vi "HelpDialog.vi"(8 "REPL Name":string, 9 "CodeRef":refnum<vi>, 11 "Microprocessor in":T1) -> (3 "Microprocessor out":T1)   [LabVIEW 2016]
uses:
  <userlib>/MicroPython/VIs/ColorText/Code.xctl
  <vilib>/Platform/browser.llb/Open URL in Default Browser (string).vi
panel:
  in  "Examples":string(tree)
  in  "Processor":u16(ring) items=["Generic", "Huzzah", "MicroBit", "OpenMV", "Pololu", "PyBoard", "PyCom"]
  in  "Copy":bool
  out "Code":string(xcontrol)
  # "If things do not work:\n1. check that you have NI-VISA installed"
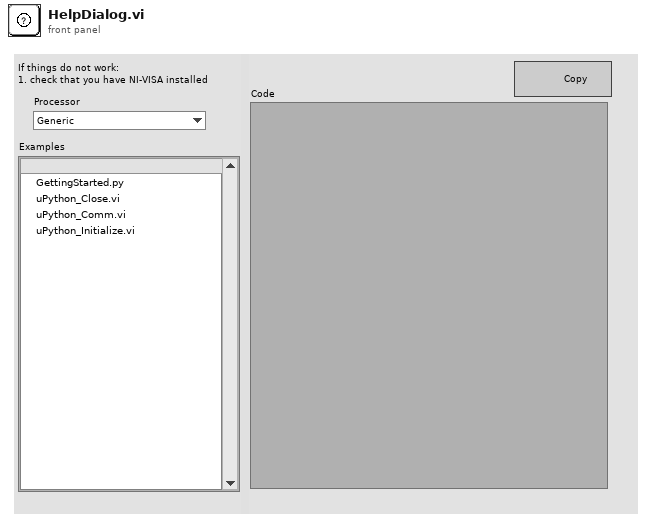
[diagram p1: front panel]
types:
  T1 = cluster{"VISA Refnum in":refnum<visa-resource-name>, "Python Code":string}
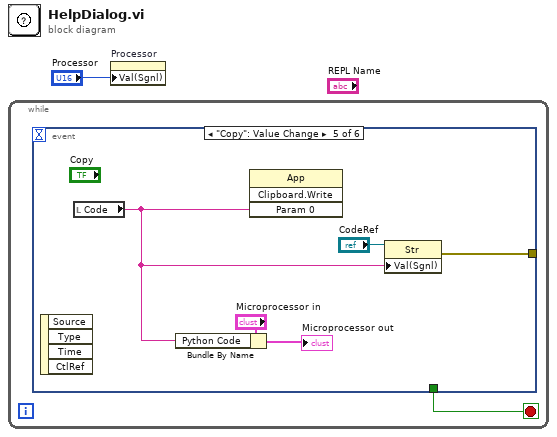
[diagram p0: block diagram]
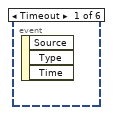
[diagram p2: hidden frame]
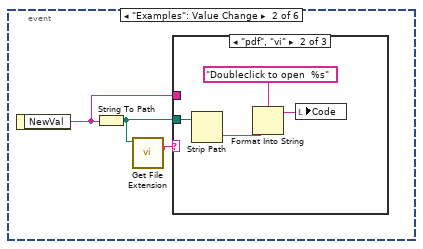
[diagram p3: hidden frame]
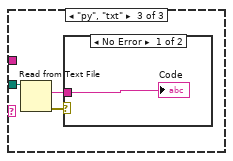
[diagram p5: hidden frame]
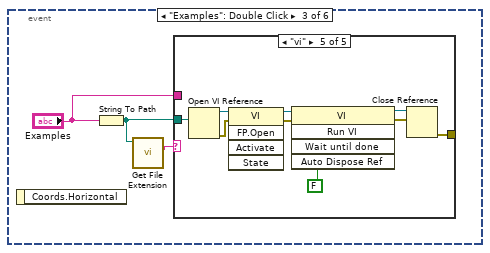
[diagram p7: hidden frame]
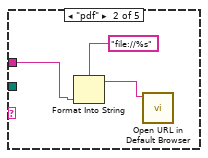
[diagram p9: hidden frame]
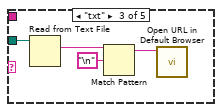
[diagram p10: hidden frame]
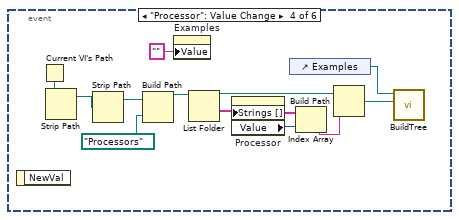
[diagram p12: hidden frame]
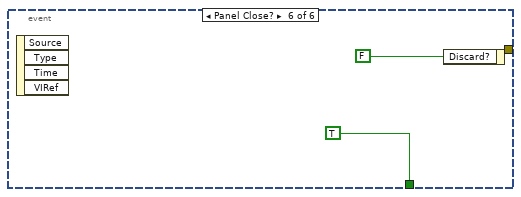
[diagram p13: hidden frame]
diagram:
  n1 = while {
    stop <- w2 stop-if-true
    n2 = event shown="[4] \"Copy\": Value Change" {
      selector: _ -> [_ _ _ _ _ _]
      dyn-events: _ -> [_ _ _ _ _ _]
      timeout: _ -> [_ _ _ _ _ _]
      tunnel: [_ _ _ _ _ TRUE ("Discard?")] -> w2
      tunnel: [_ _ _ _ w46 _] -> _
      event Timeout {
        n3 = event-data() -> ()  [unwired: 1 in, 3 out]
      }
      event "Examples": Value Change {
        n4 = event-data() -> ("NewVal"=w3:string)  [unwired: 1 in]
        n5 = String To Path(string=w3) -> (path=w5:path)
        n6 = call <vilib>:"Get File Extension.vi"("file"=w5) -> ("lowercase file extension"=w4:string)  [unwired: 6 in, 4 out]
        n7 = case shown="\"pdf\", \"vi\"" w4 {
          tunnel: w5 -> [_ w7 w10]
          tunnel: w3 -> [_ _ _]
          frame Default {
          }
          frame "pdf", "vi" {
            n8 = Strip Path(path=w7) -> (name=w6:string)  [unwired: 1 out]
            n9 = Format Into String(format string="Doubleclick to open  %s", w6) -> (resulting string=w8:string)  [unwired: 2 in, 1 out]
            n10 = local write "Code"(w8) -> ()
          }
          frame "py", "txt" {
            n11 = Read from Text File(file (use dialog)=w10) -> (text=w12:string, error out=w11:errorcluster)  [unwired: 3 in, 2 out]
            n12 = case shown="No Error" w11 {
              tunnel: w12 -> [w13 _]
              frame No Error {
                "Code" <- w13
              }
              frame Error {
              }
            }
          }
        }
      }
      event "Examples": Double Click {
        n13 = event-data() -> ()  [unwired: 1 in, 1 out]
        n14 = String To Path(string="Examples") -> (path=w16:path)
        n15 = call <vilib>:"Get File Extension.vi"("file"=w16) -> ("lowercase file extension"=w15:string)  [unwired: 6 in, 4 out]
        n16 = case shown="\"vi\"" w15 {
          tunnel: w16 -> [_ _ w23 _ w32]
          tunnel: "Examples" -> [_ w18 _ _ _]
          tunnel: [_ _ _ _ w29] -> _
          frame Default {
          }
          frame "pdf" {
            n17 = Format Into String(format string="file://%s", w18) -> (resulting string=w17:string)  [unwired: 2 in, 1 out]
            n18 = call-poly <vilib>:"Open URL in Default Browser.vi"("URL"=w17) -> ()  [unwired: 5 in, 2 out]
          }
          frame "txt" {
            n19 = Read from Text File(file (use dialog)=w23) -> (text=w22:string)  [unwired: 3 in, 3 out]
            n20 = Match Pattern(string=w22, regular expression="\n") -> (before substring=w20:string)  [unwired: 1 in, 3 out]
            n21 = call-poly <vilib>:"Open URL in Default Browser.vi"("URL"=w20) -> ()  [unwired: 5 in, 2 out]
          }
          frame "py" {
          }
          frame "vi" {
            n22 = Open VI Reference(vi path=w32) -> (vi reference=w31:refnum<vi>, error out=w30:errorcluster)  [unwired: 5 in]
            n23 = invoke class="VI" method="FP.Open"(reference=w31, error in=w30) -> (reference out=w28:refnum<vi>, error out=w27:errorcluster)  [unwired: 3 in, 3 out]
            n24 = invoke class="VI" method="Run VI"(reference=w28, error in=w27, "Wait until done"=FALSE ("Wait Until Done")) -> (reference out=w26:refnum<vi>, error out=w25:errorcluster)  [unwired: 2 in, 3 out]
            n25 = Close Reference(reference=w26, error in (no error)=w25) -> (error out=w29:errorcluster)
          }
        }
      }
      event "Processor": Value Change {
        n26 = event-data() -> ()  [unwired: 1 in, 1 out]
        n27 = Current VI's Path() -> (path=w35:path)
        n28 = Strip Path(path=w35) -> (stripped path=w37:path)  [unwired: 1 out]
        n29 = Strip Path(path=w37) -> (stripped path=w36:path)  [unwired: 1 out]
        n30 = Build Path(base path=w36, name or relative path=path "Processors") -> (appended path=w38:path)
        n31 = property on="Examples" class="Tree (strict)"("Value"="" ("Eamples")) -> ()  [unwired: 2 in, 2 out]
        n32 = List Folder(path=w38) -> (path out=w42:path, folder names=w39:string[])  [unwired: 3 in, 2 out]
        n33 = property on="Processor" class="Ring (strict)"("Strings []"=w39) -> ("Value"=w40:u16)  [unwired: 2 in, 2 out]
        n34 = control-ref of="Examples"() -> (w44:refnum<vi>)
        n35 = Index Array(array=w39, index=w40) -> (element=w41:string)
        n36 = Build Path(base path=w42, name or relative path=w41) -> (appended path=w43:path)
        n37 = call <userlib>:"BuildTree.vi"("appended path"=w43, "TreeControl in"=w44) -> ()  [unwired: 10 in]
      }
      event "Copy": Value Change {
        n38 = event-data() -> ()  [unwired: 1 in, 4 out]
        n39 = local read "Code"() -> (w48:string)
        n40 = Bundle By Name(cluster="Microprocessor in", "Python Code"=w48) -> (→"Microprocessor out":T1)
        n41 = invoke class="App" method="Clipboard.Write"("Param 0"=w48) -> ()  [unwired: 3 in, 4 out]
        n42 = property class="Str"(reference="CodeRef", "Val(Sgnl)"=w48) -> (error out=w46:errorcluster)  [unwired: 1 in, 1 out]
      }
      event Panel Close? {
        n43 = event-data() -> ()  [unwired: 1 in, 4 out]
        n44 = event-data("Discard?"=FALSE) -> ()  [unwired: 1 in, 1 out]
      }
    }
  }
  n45 = property on="Processor" class="Ring (strict)"("Val(Sgnl)"="Processor") -> ()  [unwired: 2 in, 2 out]
